vi "Save bimorph data.vi"(8 "Comments":string, 9 "Front panel settings":dbl[](array[numeric]), 10 "Data":dbl[](array[numeric]) format="%0.2f", 11 "New file?":bool) -> (3 "File path":path)   [LabVIEW 2010]
uses:
  <vilib>/Utility/file.llb/Write To Spreadsheet File (DBL).vi
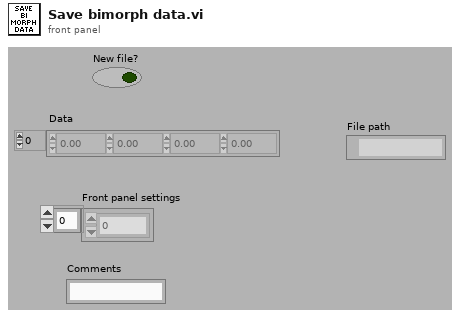
[diagram p1: front panel]
types:
  T1 = enum16{"open", "replace", "create", "open or create", "replace or create", "replace or create with confirmation"}
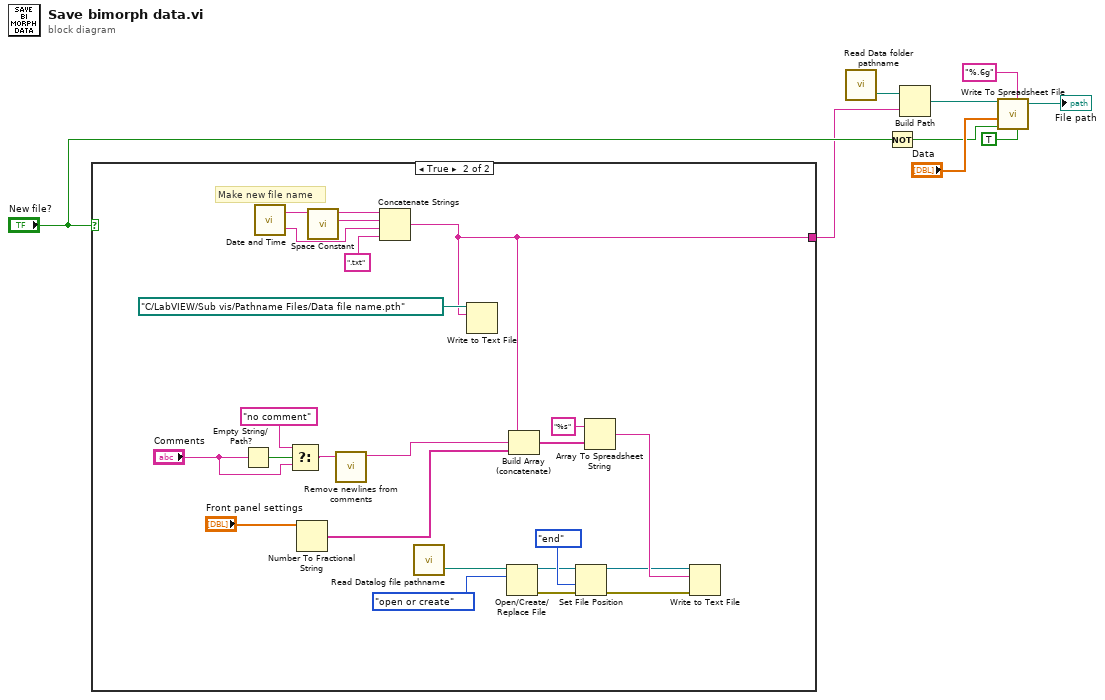
[diagram p0: block diagram]
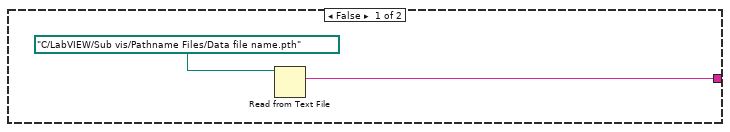
[diagram p2: hidden frame]
diagram:
  n1 = case shown="True" "New file?" {
    tunnel: [w10 w14] -> w2
    frame False {
      n2 = Read from Text File(file (use dialog)=path "C:/LabVIEW/Sub vis/Pathname Files/Data file name.pth") -> (text=w10:string)  [unwired: 3 in, 3 out]
    }
    frame True {
      # "Make new file name"
      n3 = Empty String/Path?(string/path="Comments") -> (empty?=w23:bool)
      n4 = call "Date and Time.vi"() -> ("Time string."=w30:string, "Date string."=w32:string)
      n5 = Select(t="no comment" ("format string"), s=w23, f="Comments") -> (s? t:f=w13:string)
      n6 = Number To Fractional String(number="Front panel settings") -> (F-format string=w26:string[])  [unwired: 3 in]
      n7 = call <vilib>:"Space Constant.vi"() -> ("String"=w31:string)
      n8 = call "Remove newlines from comments.vi"("Comments IN"=w13) -> ("Comments OUT"=w12:string)  [unwired: 10 in]
      n9 = Concatenate Strings(w32, w31, w30, ".txt") -> (w14:string)
      n10 = call "Read Datalog file pathname.vi"() -> ("Datalog file pathname."=w15:path)  [unwired: 1 out]
      n11 = Write to Text File(file (use dialog)=path "C:/LabVIEW/Sub vis/Pathname Files/Data file name.pth", text=w14) -> ()  [unwired: 2 in, 3 out]
      n12 = Open/Create/Replace File(file path (use dialog)=w15, operation (0:open)=T1."open or create") -> (refnum out=w17:refnum<file>, error out=w18:errorcluster)  [unwired: 4 in, 1 out]
      n13 = Build Array (concatenate)(w14, w12, w26) -> (w27:string[])
      n14 = Set File Position(refnum=w17, from (0:start)=enum16{"start", "end", "current"}."end", error in=w18) -> (refnum out=w20:refnum<file>, error out=w21:errorcluster)  [unwired: 1 in]
      n15 = Array To Spreadsheet String(array=w27, 3:"%s" ("format string")) -> (spreadsheet string=w29:string)  [unwired: 1 in]
      n16 = Write to Text File(file (use dialog)=w20, text=w29, error in=w21) -> ()  [unwired: 1 in, 3 out]
    }
  }
  n17 = call "Read Data folder pathname.vi"() -> ("Data folder pathname."=w9:path)  [unwired: 1 out]
  n18 = Not(x="New file?") -> (.not. x?=w3:bool)
  n19 = Build Path(base path=w9, name or relative path=w2) -> (appended path=w8:path)
  n20 = call-poly <vilib>:"Write To Spreadsheet File.vi"("transpose? (no:F)"=TRUE, "format (%.3f)"="%.6g", "append to file? (new file:F)"=w3, "1D data"="Data", "file path (dialog if empty)"=w8) -> ("new file path (Not A Path if cancelled)"=→"File path":path)  [unwired: 3 in]
